vi "Contingency_Matrix.vi"(8 "error in (no error)":errorcluster caption="entrée d'erreur (pas d'erreur)", 9 "labels_pred":string[][](array[string]), 10 "labels_true":string[][](array[string]), 11 "contingency_matrix":cluster{"eps":string, "sparse":bool}={"eps"="None", "sparse"=FALSE}) -> (0 "error out":errorcluster caption="sortie d'erreur", 3 "Data":T1)   [LabVIEW 2020]
doc: "Build a contingency matrix describing the relationship between labels.\n\nParameters :\n\n- labels_true : int array, shape = [n_samples]\nGround truth class labels to be used as a reference\n\n- labels_pred : array-like of shape (n_samples,)\nCluster labels to evaluate\n\n- eps : None or float, optional.\nIf a float, that value is added to all values in the contingency matrix. This helps to stop NaN propagation. If None, nothing is adjusted.\n\n- sparse : boolean, optional.\nIf True, return a sparse CSR continency matrix. If eps is not None, and sparse is True, will throw ValueError.\n\n\nReturns :\n\n- contingency : {array-like, sparse}, shape=[n_classes_true, n_classes_pred]\nMatrix such that is the number of samples in true class and in predicted class . If eps is None, the dtype of this array will be integer. If eps is given, the dtype will be float. Will be a scipy.sparse.csr_matrix if sparse=True."
uses:
  Contingency_Matrix.lvclass
panel:
  out "Contingency_Matrix.lvclass":refnum<class "Contingency_Matrix.lvclass">
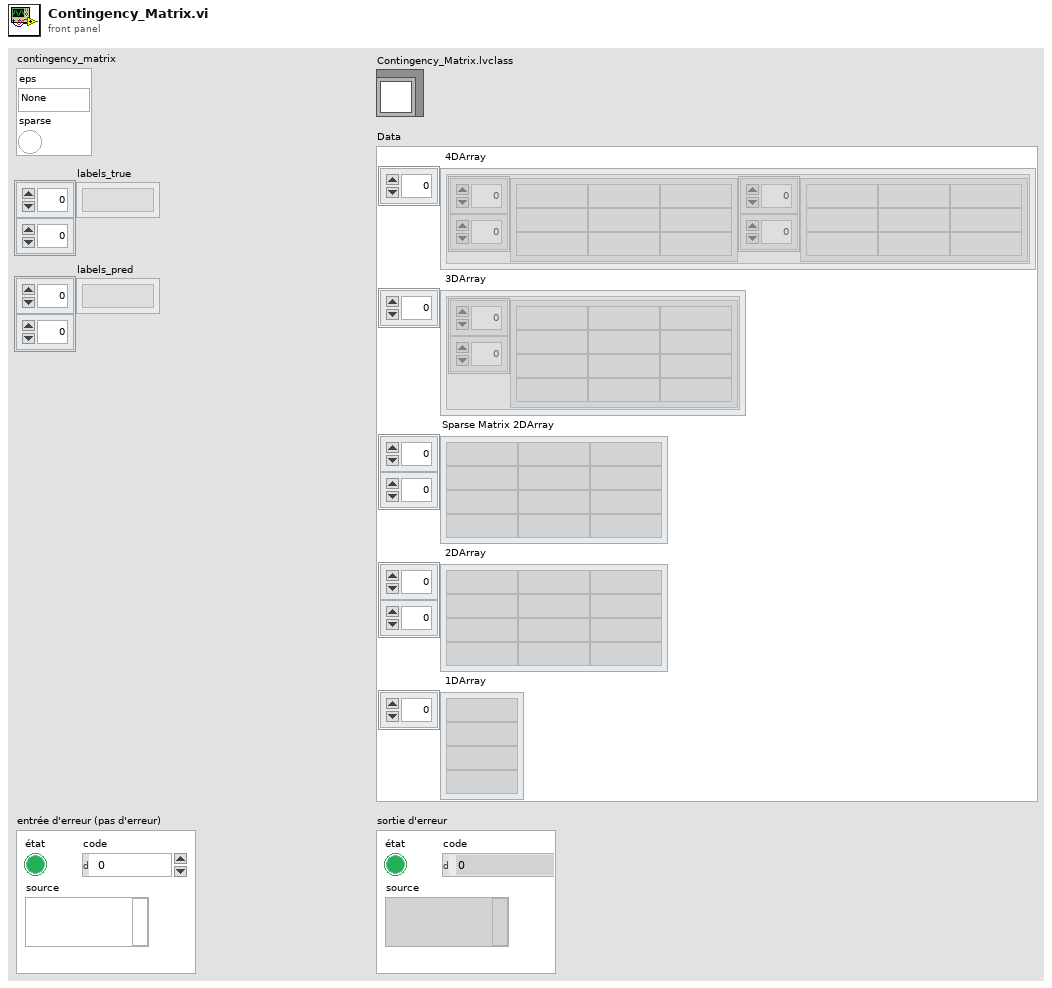
[diagram p1: front panel]
types:
  T1 = cluster{" 4DArray":cluster{"1":string[][], "2":string[][]}[], " 3DArray":cluster{"Tableau":string[][]}[], "Sparse Matrix 2DArray":string[][], " 2DArray":string[][], " 1DArray":string[]}
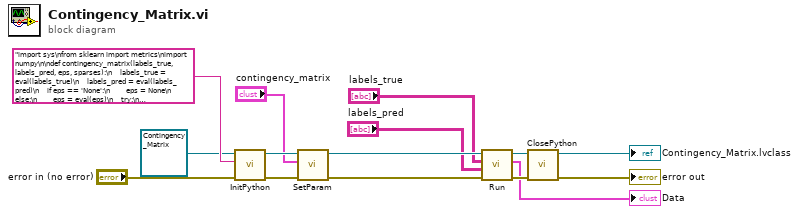
[diagram p0: block diagram]
diagram:
  n1 = call-dynamic "InitPython.vi"("error in (no error)"="error in (no error)", "Python Instruction"="import sys\nfrom sklearn import metrics\nimport numpy\n\ndef contingency_matrix(labels_true, labels_pred, eps, sparses):\n    labels_true = eval(labels_true)\n    labels_pred = eval(labels_pred)\n    if eps == 'None':\n        eps = None\n    else:\n        eps = eval(eps)\n    try:\n        contingency_matrix = metrics.cluster.contingency_matrix(labels_true, labels_pred, eps, sparses)\n        dtype = type(contingency_matrix)\n        if dtype == numpy.ndarray:\n            contingency_matrix = contingency_matrix.tolist()\n            return str(contingency_matrix)\n        else:\n            Mat = contingency_matrix.tocoo()\n            return str(list(zip(Mat.row, Mat.col, Mat.data)))\n        return dtype\n    except:\n        erreur = sys.exc_info()\n        typerr = u\"%s\" % (erreur[0])\n        typerr = typerr[typerr.find(\"'\")+1:typerr.rfind(\"'\")]\n        msgerr = u\"%s\" % (erreur[1])\n        message = str('/!\\\\ {0} : {1}'. format(typerr,msgerr))\n        return message", "Scikit-learn en entrée"=refnum<class "Contingency_Matrix.lvclass"> refnum ("Contingency_Matrix.lvclass")) -> ("error out"=w8:errorcluster, "Scikit-learn en sortie"=w10:refnum<class "Contingency_Matrix.lvclass">)  [unwired: 7 in]
  n2 = call-dynamic "SetParam.vi"("error in (no error)"=w8, "contingency_matrix"="contingency_matrix", "Contingency_Matrix.lvclass"=w10) -> ("error out"=w6:errorcluster, "Contingency_Matrix.lvclass"=w7:refnum<class "Contingency_Matrix.lvclass">)  [unwired: 7 in]
  n3 = call-dynamic "Run.vi"("error in (no error)"=w6, "labels_pred"="labels_pred", "labels_true"="labels_true", "Contingency_Matrix.lvclass"=w7) -> ("error out"=w11:errorcluster, "Data"=→"Data":T1, "Contingency_Matrix.lvclass"=w12:refnum<class "Contingency_Matrix.lvclass">)  [unwired: 5 in]
  n4 = call-dynamic "ClosePython.vi"("error in (no error)"=w11, "Scikit-learn en entrée"=w12) -> ("error out"=→"error out":errorcluster, "Scikit-learn en sortie"=→"Contingency_Matrix.lvclass":refnum<class "Contingency_Matrix.lvclass">)  [unwired: 8 in]
